vi "ChannelType_2D-Array-U32_Color.vi"(9 "error in":errorcluster, 11 "Array in":u32[][](array[numeric])) -> (1 "error out":errorcluster, 2 "ChannelType":u8, 3 "Array out":u32[][](array[numeric]))   [LabVIEW 2020, in "OpenLvVision_OpenCv.lvlib"]
uses:
  OpenLvVision_OpenCv.lvlib
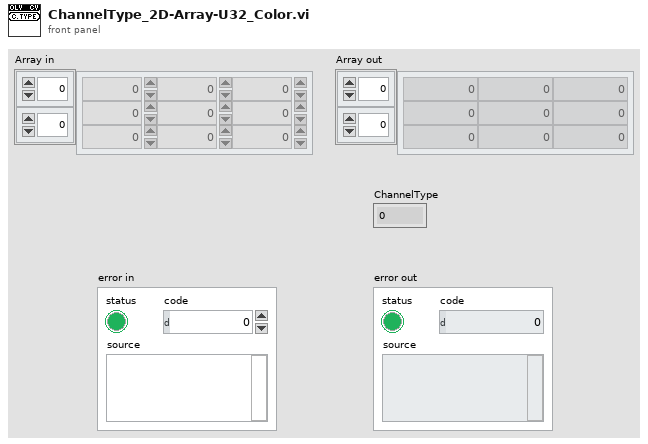
[diagram p1: front panel]
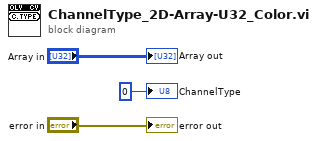
[diagram p0: block diagram]
diagram:
  "error out" <- "error in"
  "Array out" <- "Array in"
  "ChannelType" <- u8 0
